vi "Read.vi"(8 "error in (no error)":errorcluster, 10 "Numeric Control":i32, 11 "file path (dialog if empty)":path=path "D:/LABView/Kinect_Projekt/Controls/RGB_Table.csv") -> ()   [LabVIEW 2017]
uses:
  <vilib>/Utility/file.llb/Read Delimited Spreadsheet (DBL).vi
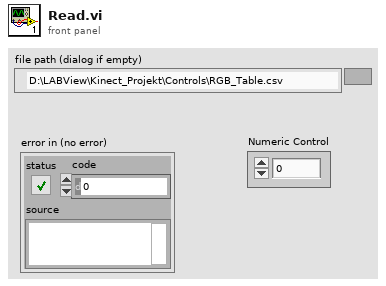
[diagram p1: front panel]
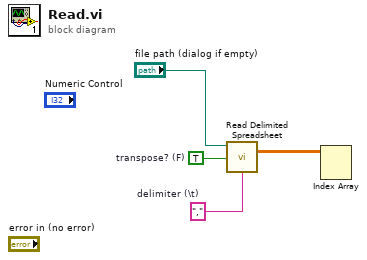
[diagram p0: block diagram]
diagram:
  w3 = TRUE  # transpose? (F)
  w4 = ","  # delimiter (\t)
  n1 = call-poly <vilib>:"Read Delimited Spreadsheet.vi"("file path (dialog if empty)"="file path (dialog if empty)", "transpose? (F)"=w3, "delimiter (\\t)"=w4) -> ("all rows"=w1:dbl[][])  [unwired: 7 in, 5 out]
  n2 = Index Array(array=w1) -> ()  [unwired: 2 in, 1 out]
